vi "Error Event.vi"(2 "error in (no error)":errorcluster, 4 "Enum":enum16{"Create", "Default", "Destroy"}(ring)=enum."Default") -> (5 "Event Registration Refnum":refnum<event-registration>, 6 "error out":errorcluster)   [LabVIEW 2018]
doc: "Creates a user defined event for the error cluster. An input error will trigger the event. Error out will be cleared unless the user event generates an error."
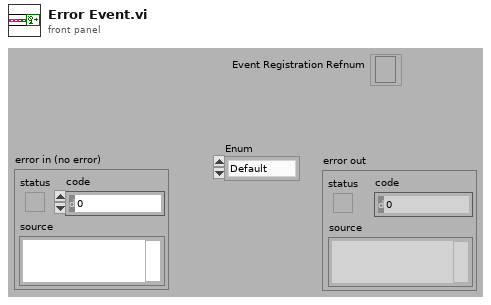
[diagram p1: front panel]
types:
  T1 = cluster{"call chain":string[], "error in (no error)":errorcluster}
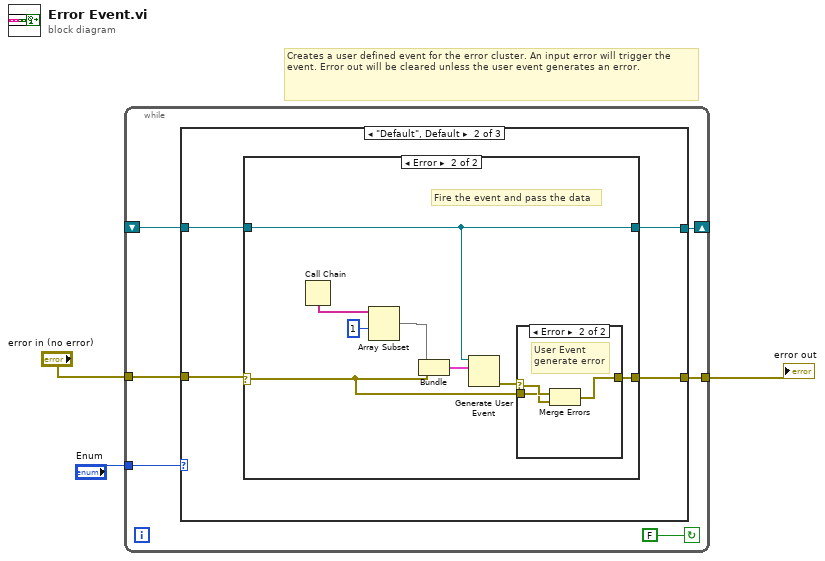
[diagram p0: block diagram]
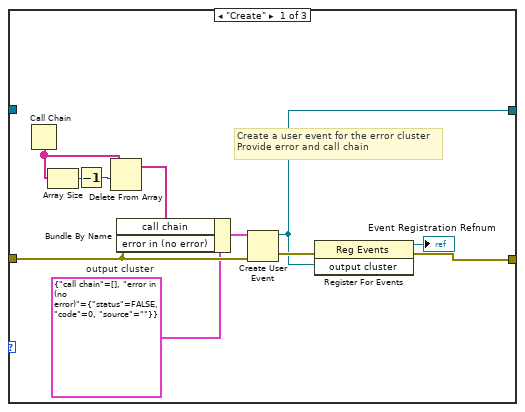
[diagram p2: hidden frame]
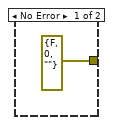
[diagram p4: hidden frame]
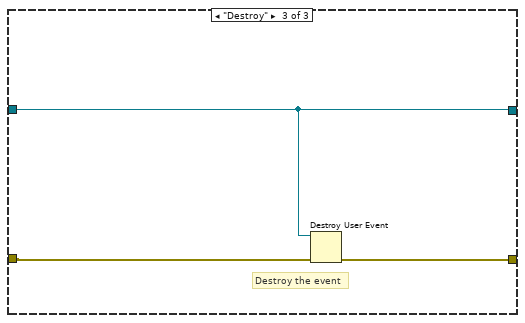
[diagram p5: hidden frame]
diagram:
  # "Creates a user defined event for the error cluster. An input error will trigger the event. Error out will be cleared unless the user event generates an error."
  n1 = while {
    shift-right: [w5] -> _
    shift-left: _ -> [w7]
    tunnel: "Enum" -> [w8]
    tunnel: "error in (no error)" -> [w6]
    tunnel: [w4] -> w1
    stop <- FALSE continue-if-true
    n2 = case shown="\"Default\", Default" w8 {
      tunnel: [w19 w22 w41] -> w5
      tunnel: w7 -> [_ w23 w41]
      tunnel: w6 -> [w16 w24 w39]
      tunnel: [w18 w21 w40] -> w4
      frame "Create" {
        w10 = T1 {"call chain"=[], "error in (no error)"={"status"=FALSE, "code"=0, "source"=""}}  # output cluster
        # "Create a user event for the error cluster\nProvide error and call chain"
        n3 = Call Chain() -> (call chain=w13:string[])
        n4 = Array Size(array=w13) -> (size(s)=w15:i32)
        n5 = Decrement(x=w15) -> (x-1=w14:i32)
        n6 = Delete From Array(array=w13, length=w14) -> (array with subset deleted=w11:string[])  [unwired: 1 in, 1 out]
        n7 = Bundle By Name(cluster=w10, "call chain"=w11, "error in (no error)"=w16) -> (w17:T1)
        n8 = Create User Event(user event datatype=w17, error in=w16) -> (user event=w19:refnum<user-event>, error out=w20:errorcluster)
        n9 = register-events(error in=w20, w19) -> (reference out=→"Event Registration Refnum":refnum<event-registration>, error out=w18:errorcluster)  [unwired: 1 in]
      }
      frame "Default", Default {
        n10 = case shown="Error" w24 {
          selector: w24 -> [w25 w31]
          tunnel: w23 -> [w26 w34]
          tunnel: [w26 w34] -> w22
          tunnel: [w25 w32] -> w21
          frame No Error {
          }
          frame Error {
            # "Fire the event and pass the data"
            n11 = Call Chain() -> (call chain=w29:string[])
            n12 = Array Subset(array=w29, index=1) -> (w28:string[])  [unwired: 1 in]
            n13 = Bundle(w28, "error IO"=w31) -> (w30:cluster{string[], "error IO":errorcluster})  [unwired: 1 in]
            n14 = Generate User Event(user event=w34, event data cluster=w30) -> (error out=w33:errorcluster)  [unwired: 2 in, 1 out]
            n15 = case shown="Error" w33 {
              selector: w33 -> [_ w38]
              tunnel: [errorcluster {"status"=FALSE, "code"=0, "source"=""} ("error out") w36] -> w32
              tunnel: w31 -> [_ w37]
              frame No Error {
              }
              frame Error {
                # "User Event\ngenerate error"
                n16 = Merge Errors(w38, w37) -> (w36:errorcluster)
              }
            }
          }
        }
      }
      frame "Destroy" {
        # "Destroy the event"
        n17 = Destroy User Event(user event=w41, error in=w39) -> (error out=w40:errorcluster)
      }
    }
  }
  "error out" <- w1
